vi "automatic_step_state.vi"(7 "transition_queue":refnum<queue>, 8 "error in (no error)":errorcluster, 10 "data":variant, 11 "recipe_data":variant) -> (0 "error out":errorcluster)   [LabVIEW 2015, in "lv-recipe-machine.lvlib" / "example_02.lvlib"]
uses:
  example_02.lvlib
  public/_controls/transition.ctl
  _controls/customer.ctl
  lv-recipe-machine.lvlib
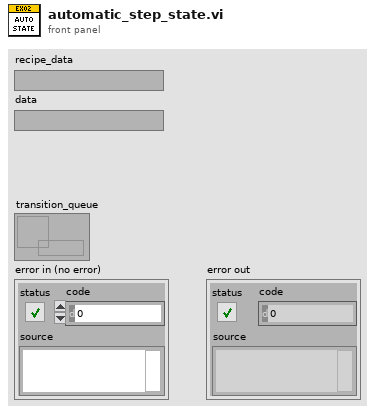
[diagram p1: front panel]
types:
  T1 = typedef "lv-recipe-machine.lvlib/example_02.lvlib/customer.ctl" = cluster{"first_name":string, "last_name":string, "address_1":string, "address_2":string, "city":string, "state":string, "zip_code":string}
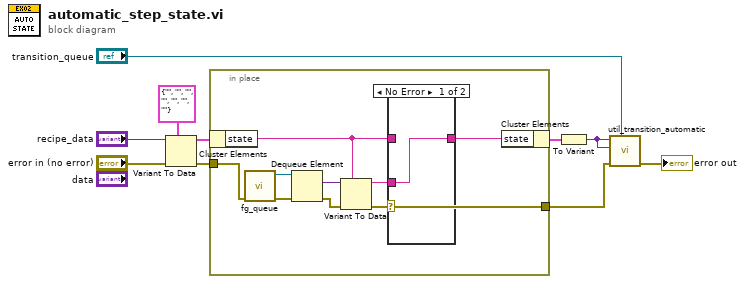
[diagram p0: block diagram]
diagram:
  n1 = Variant To Data(error in="error in (no error)", type=T1 {"first_name"="", "last_name"="", "address_1"="", "address_2"="", "city"="", "state"="", "zip_code"=""} ("customer"), Variant="recipe_data") -> (data=w5:T1, error out=w2:errorcluster)
  n2 = in-place {
    in-place-border: w2 -> [w17]
    in-place-border: [w14] -> w1
    n3 = in-place-cluster #1(w5) -> ("state"=w15:string)
    n4 = call "fg_queue.vi"("error in (no error)"=w17) -> ("error out"=w18:errorcluster, "queue out"=w19:refnum<queue>)  [unwired: 9 in]
    n5 = Dequeue Element(queue=w19, error in (no error)=w18) -> (element=w11:variant, error out=w16:errorcluster)  [unwired: 1 in, 2 out]
    n6 = Variant To Data(error in=w16, type=w15, Variant=w11) -> (data=w13:string, error out=w14:errorcluster)
    n7 = case shown="No Error" w14 {
      tunnel: w15 -> [_ w21]
      tunnel: w13 -> [w20 _]
      tunnel: [w20 w21] -> w12
      frame No Error {
      }
      frame Error {
      }
    }
    n8 = in-place-cluster #1("state"=w12) -> (w4:T1)
  }
  n9 = To Variant(anything=w4) -> (Variant=w3:variant)
  n10 = call "util_transition_automatic.vi"("transition_queue"="transition_queue", "error in (no error)"=w1, "data"=w3, "recipe_data"=w3) -> ("error out"=→"error out":errorcluster)  [unwired: 7 in]
